vi "Write Init Data.vi"() -> ()   [LabVIEW 2017]
uses:
  Type Definitions/DB Record.ctl
panel:
  in  "DB Record":T1 {"Balance" format="%.2f"; "Account" format="%05d"}
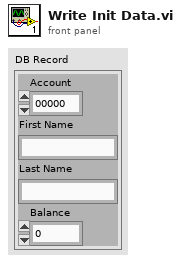
[diagram p1: front panel]
types:
  T1 = typedef "DB Record.ctl" = cluster{"Account":i32, "First Name":string, "Last Name":string, "Balance":fxp<+/-,64,35>}
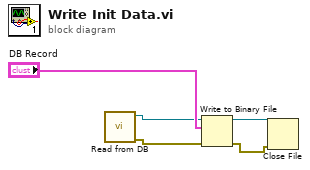
[diagram p0: block diagram]
diagram:
  n1 = call "Read from DB.vi"() -> ("error out"=w3:errorcluster, "refnum out"=w4:refnum<file>)  [unwired: 9 in, 1 out]
  n2 = Write to Binary File(file (use dialog)=w4, data="DB Record", error in=w3) -> (refnum out=w2:refnum<file>, error out=w1:errorcluster)  [unwired: 3 in, 1 out]
  n3 = Close File(refnum=w2, error in=w1) -> ()  [unwired: 2 out]
